vi "ErrorHandlerUpdate.vi"(11 "Small Input Cluster":T1(array[cluster])) -> (2 "Unsorted Timestamps":dbl[](array[numeric]), 3 "Full Error Cluster":T1(array[cluster]))   [LabVIEW 2013]
uses:
  GlobalErrorCluster.vi
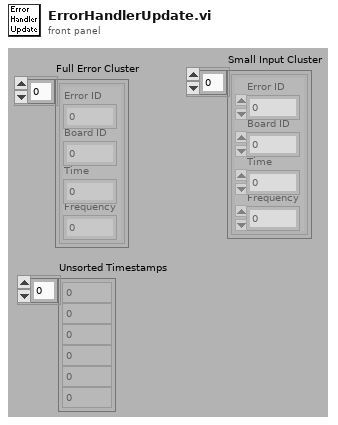
[diagram p1: front panel]
types:
  T1 = cluster{"Error ID":i32, "Board ID":i32, "Time":u32, "Frequency":i32}[]
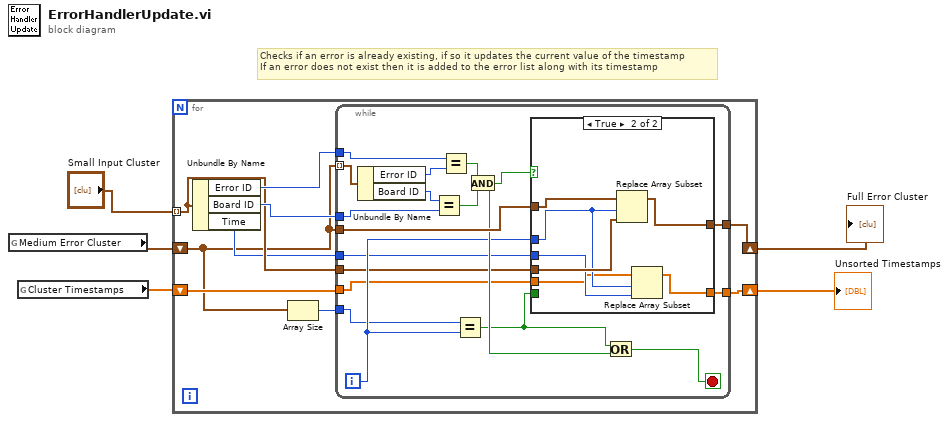
[diagram p0: block diagram]
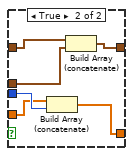
[diagram p3: hidden frame]
diagram:
  # "Checks if an error is already existing, if so it updates the current value of the timestamp\nIf an error does not exist then it is added to the error list along with its timestamp"
  n1 = global read "GlobalErrorCluster.vi" "Medium Error Cluster"() -> (w2:T1)
  n2 = global read "GlobalErrorCluster.vi" "Cluster Timestamps"() -> (w3:dbl[])
  n3 = for {
    tunnel: "Small Input Cluster" -> [w11] mode=indexing
    shift-right: [w7] -> w1
    shift-left: w3 -> [w8]
    shift-right: [w10] -> w4
    shift-left: w2 -> [w6]
    n4 = Unbundle By Name(w11) -> ("Error ID"=w14:i32, "Board ID"=w13:i32, "Time"=w9:u32)
    n5 = Array Size(array=w6) -> (size(s)=w12:i32)
    n6 = while {
      tunnel: w6 -> [w32] mode=indexing
      tunnel: w14 -> [w22]
      tunnel: w13 -> [w30]
      tunnel: w6 -> [w27]
      tunnel: w12 -> [w15]
      tunnel: w11 -> [w24]
      tunnel: [w20] -> w10
      tunnel: w9 -> [w18]
      tunnel: [w17] -> w7
      tunnel: w8 -> [w16]
      i -> [w25]
      stop <- w21 stop-if-true
      n7 = Unbundle By Name(w32) -> ("Error ID"=w23:i32, "Board ID"=w31:i32)
      n8 = Equal?(x=w31, y=w30) -> (x = y?=w29:bool)
      n9 = Equal?(x=w22, y=w23) -> (x = y?=w28:bool)
      n10 = Equal?(x=w15, y=w25) -> (x = y?=w19:bool)
      n11 = And(x=w29, y=w28) -> (x .and. y?=w26:bool)
      n12 = case shown="True" w26 {
        tunnel: w25 -> [_ w51]
        tunnel: w27 -> [w38 w54]
        tunnel: w24 -> [w37 w53]
        tunnel: [w36 w52] -> w20
        tunnel: w19 -> [w39 _]
        tunnel: w18 -> [w35 w50]
        tunnel: [w34 w49] -> w17
        tunnel: w16 -> [w33 w48]
        frame False {
          n13 = case shown="False" w39 {
            tunnel: w38 -> [w41 w47]
            tunnel: w37 -> [_ w46]
            tunnel: [w41 w45] -> w36
            tunnel: w35 -> [_ w44]
            tunnel: [w40 w43] -> w34
            tunnel: w33 -> [w40 w42]
            frame False {
            }
            frame True {
              n14 = Build Array (concatenate)(w42, w44) -> (w43:dbl[])
              n15 = Build Array (concatenate)(w47, w46) -> (w45:T1)
            }
          }
        }
        frame True {
          n16 = Replace Array Subset(array=w54, new element=w53, index=w51) -> (w52:T1)
          n17 = Replace Array Subset(array=w48, new element=w50, index=w51) -> (w49:dbl[])
        }
      }
      n18 = Or(x=w19, y=w26) -> (x .or. y?=w21:bool)
    }
  }
  "Full Error Cluster" <- w4
  "Unsorted Timestamps" <- w1
